vi "PC_Main_SequenceEditor_AddNewStep.vi"() -> ()   [LabVIEW 2010]
uses:
  Ctls/StepData.ctl
panel:
  in  "Tab Control":enum32{"POC", "SCOPE", "DMM", "FDEN"}(tab)
  in  "Parameter":dbl
  out "Enable":bool
  out "new element/subarray":T1
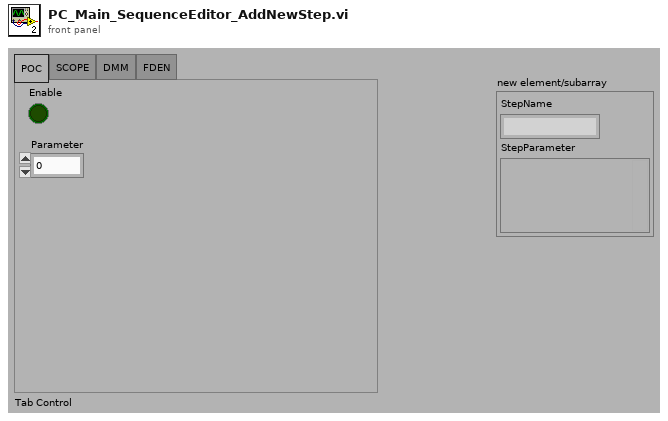
[diagram p1: front panel]
types:
  T1 = typedef "StepData.ctl" = cluster{"StepName":string, "StepParameter":variant}
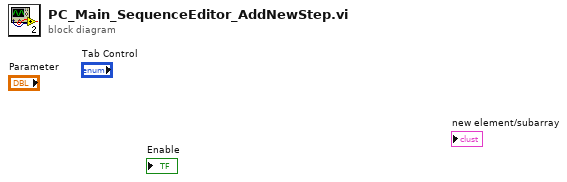
[diagram p0: block diagram]
diagram:
